vi "ex_Enable.vi"(1 "Enable?":bool) -> (0 "Disabled Value":u8)   [LabVIEW 2017]
doc: "Returns a value of 0 if Enable? is TRUE, otherwise returns 2."
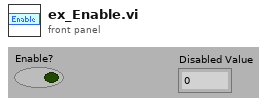
[diagram p1: front panel]
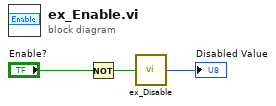
[diagram p0: block diagram]
diagram:
  n1 = Not(x="Enable?") -> (.not. x?=w2:bool)
  n2 = call <vilib>:"ex_Disable.vi"("Disable?"=w2) -> ("Disabled value"=→"Disabled Value":u8)
